vi "Write Outgoing Bytes.vi"(8 "error in (no error)":errorcluster, 10 "Bytes":u8[](array[numeric]) format="%08b", 11 "TCPConnection in":refnum<class "TCPConnection.lvclass">) -> (0 "error out":errorcluster, 3 "TCPConnection out":refnum<class "TCPConnection.lvclass">)   [LabVIEW 2013, in "MQTT_TCP.lvlib" / "TCPConnection.lvclass"]
uses:
  TCPConnection.lvclass
  TCPConnection.lvclass/TCPConnection.ctl
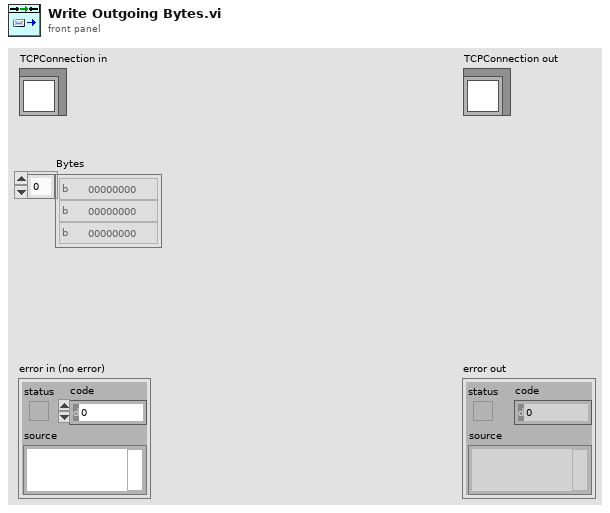
[diagram p1: front panel]
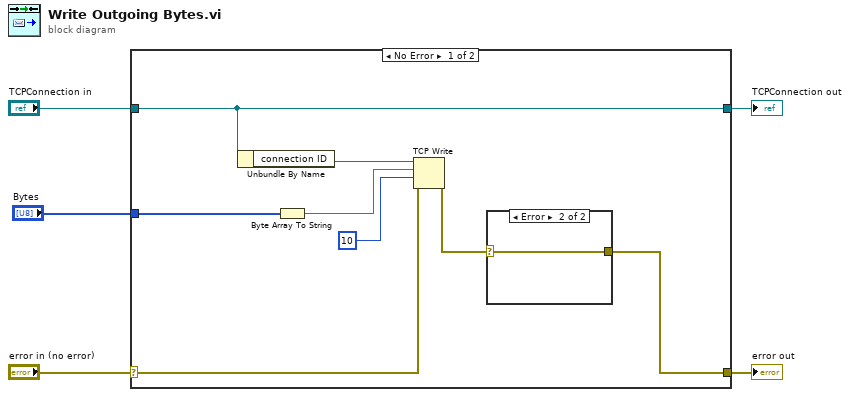
[diagram p0: block diagram]
diagram:
  n1 = case shown="No Error" "error in (no error)" {
    selector: "error in (no error)" -> [w8 w17]
    tunnel: [w6 w17] -> w4
    tunnel: [w13 w16] -> w2
    tunnel: "TCPConnection in" -> [w13 w16]
    tunnel: "Bytes" -> [w11 _]
    frame No Error {
      n2 = Unbundle By Name(w13) -> ("connection ID"=w12:refnum<k5>)
      n3 = Byte Array To String(unsigned byte array=w11) -> (string=w10:string)
      n4 = TCP Write(connection ID=w12, data in=w10, error in (no error)=w8, 9:10 ("timeout ms (25000)")) -> (error out=w7:errorcluster)  [unwired: 2 out]
      n5 = case shown="Error" w7 {
        selector: w7 -> [w14 w15]
        tunnel: [w14 w15] -> w6
        frame No Error {
        }
        frame Error {
        }
      }
    }
    frame Error {
    }
  }
  "error out" <- w4
  "TCPConnection out" <- w2
